vi "SSC DCPower Configure Sense.vi"(0 "DCPower SSC in":T2[](array[typedef]), 5 "Sense":T1=1008 items=["Local"=1008, "Remote"=1009], 11 "error in":errorcluster) -> (4 "DCPower SSC out":T2[](array[typedef]), 15 "error out":errorcluster)   [LabVIEW 2020]
doc: "This VI configures local or remote sense for the sessions."
uses:
  SSC DCPower.ctl
  <instrlib>/niDCPower/nidcpower.llb/niDCPower Sense.ctl
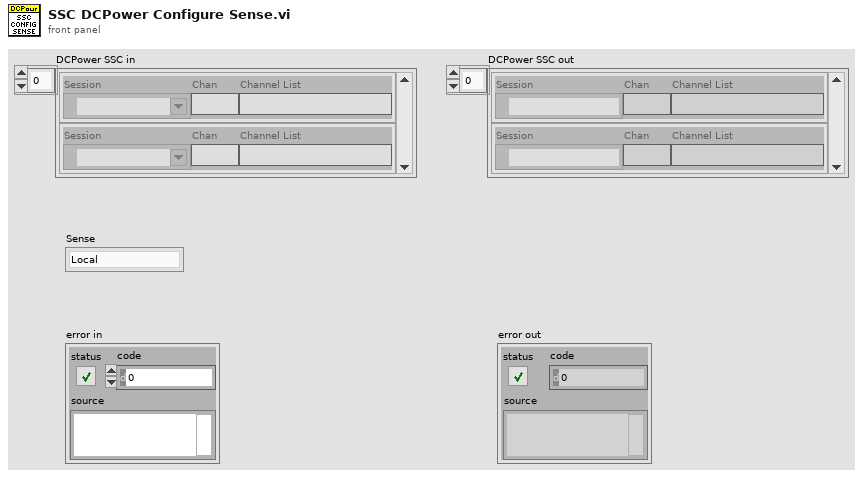
[diagram p1: front panel]
types:
  T1 = typedef "niDCPower Sense.ctl" = i32
  T2 = typedef "SSC DCPower.ctl" = cluster{"Session":refnum<k15>, "Chan":string, "Channel List":string}
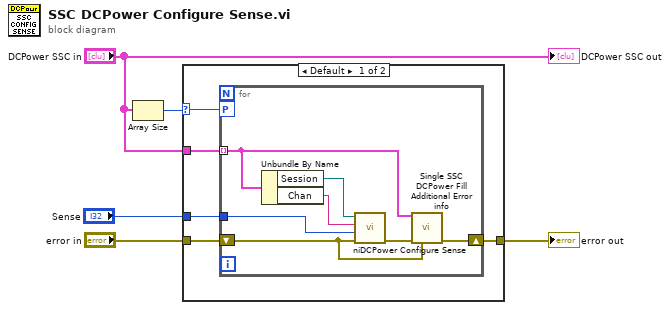
[diagram p0: block diagram]
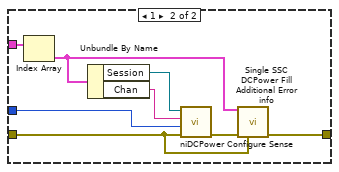
[diagram p2: hidden frame]
diagram:
  n1 = Array Size(array="DCPower SSC in") -> (size(s)=w2:i32)
  n2 = case shown="Default" w2 {
    selector: w2 -> [w7 _]
    tunnel: "error in" -> [w10 w25]
    tunnel: "Sense" -> [w9 w24]
    tunnel: [w8 w23] -> w3
    tunnel: "DCPower SSC in" -> [w6 w22]
    frame Default {
      n3 = for {
        tunnel: w6 -> [w12] mode=indexing
        tunnel: w9 -> [w16]
        workers-P: w7 -> [_]
        shift-right: [w13] -> w8
        shift-left: w10 -> [w11]
        n4 = Unbundle By Name(w12) -> ("Session"=w15:refnum<k15>, "Chan"=w14:string)
        n5 = call <instrlib>:"niDCPower Configure Sense.vi"("error in (no error)"=w11, "sense"=w16, "channel name"=w14, "instrument handle"=w15) -> ("error out"=w17:errorcluster)  [unwired: 6 in, 1 out]
        n6 = call "Single SSC DCPower Fill Additional Error info.vi"("DCPower SSC in"=w12, "error in"=w17, "previous error in"=w11) -> ("error out"=w13:errorcluster)  [unwired: 12 in]
      }
    }
    frame 1 {
      n7 = Index Array(array=w22) -> (element=w18:T2)  [unwired: 1 in]
      n8 = Unbundle By Name(w18) -> ("Session"=w20:refnum<k15>, "Chan"=w19:string)
      n9 = call <instrlib>:"niDCPower Configure Sense.vi"("error in (no error)"=w25, "sense"=w24, "channel name"=w19, "instrument handle"=w20) -> ("error out"=w21:errorcluster)  [unwired: 6 in, 1 out]
      n10 = call "Single SSC DCPower Fill Additional Error info.vi"("DCPower SSC in"=w18, "error in"=w21, "previous error in"=w25) -> ("error out"=w23:errorcluster)  [unwired: 12 in]
    }
  }
  "error out" <- w3
  "DCPower SSC out" <- "DCPower SSC in"
